vi "CANOpen NMTs.vi"(8 "error in (no error)":errorcluster, 11 "Node Ptr":T3 format="%.0x") -> (0 "error out":errorcluster)   [LabVIEW 2021, in "CANOpen Addon System Explorer.lvlib"]
uses:
  CANOpen Addon System Explorer.lvlib
  <vilib>/NI VeriStand/Custom Device API/Custom Device Item Ref.ctl
  Driver/Async VIs/CANOpen_Main/SubVIs/CanOpen_NMT_Config.ctl
  Driver/Async VIs/CANOpen_Main/SubVIs/CanOpen_NMT_Static detect.ctl
  Shared/CANOpen Addon GUID Lookup Global.vi
  <vilib>/NI VeriStand/Custom Device API/Get Item Property (Variant).vi
  <vilib>/NI VeriStand/Custom Device API/Set Item Property (Variant).vi
  <vilib>/NI VeriStand/Custom Device API/Custom Device API.lvlib
  Shared/CANOpen Addon Shared.lvlib
  Driver/CANOpen Addon Engine.lvlib
panel:
  in  "*HB NG":T1={"Mode"=enum."HB", "Update Time"=100, "Static detect in None"=enum."NG"} caption="Hearbeat and Node Guarding settings"
  in  "*Stop and Reset on Shutdown":bool=TRUE caption="Stop and Reset node on Shutdown"
  in  "*Emergency":bool=TRUE caption="Emergency enabled"
  in  "*Delay for opp. state (ms)":dbl=100.0 caption="Delay (ms) before going to run mode"
  in  "*Node init static SDO state":u16(ring)=128 caption="Inital mode before configuration" items=["start remote node"=1, "enter pre-operational"=128]
  in  "*Node run state":u16(ring)=1 caption="Mode in run state" items=["start remote node"=1, "stop remote node"=2, "enter pre-operational"=128, "reset node"=129, "reset communication"=130]
  in  "SHDocVw.IWebBrowser2":refnum<k7>(container)
  in  "Header":cluster{"Section Name":string}={"Section Name"="NMT"}
  in  "Description":string
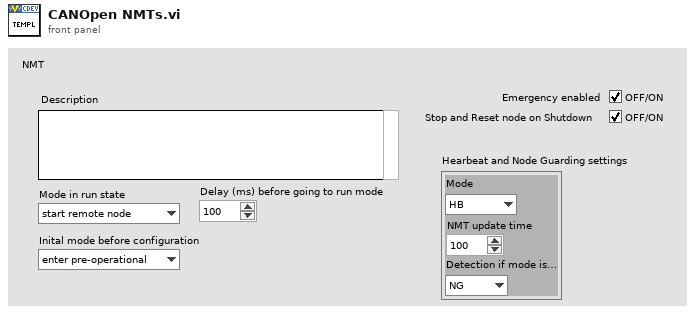
[diagram p1: front panel]
types:
  T1 = typedef "CANOpen Addon Engine.lvlib/CanOpen_NMT_Config.ctl" = cluster{"Mode":T2, "Update Time":u16, "Static detect in None":T2}
  T2 = typedef "CANOpen Addon Engine.lvlib/CanOpen_NMT_Static detect.ctl" = enum16{"None", "HB", "NG"}
  T3 = typedef "Custom Device API.lvlib/Custom Device Item Ref.ctl" = u64
  T4 = typedef "Custom Device API.lvlib/Custom Device Commands.ctl" = enum16{"Default", "Item renamed", "Shutdown", "Dynamic button pressed"}
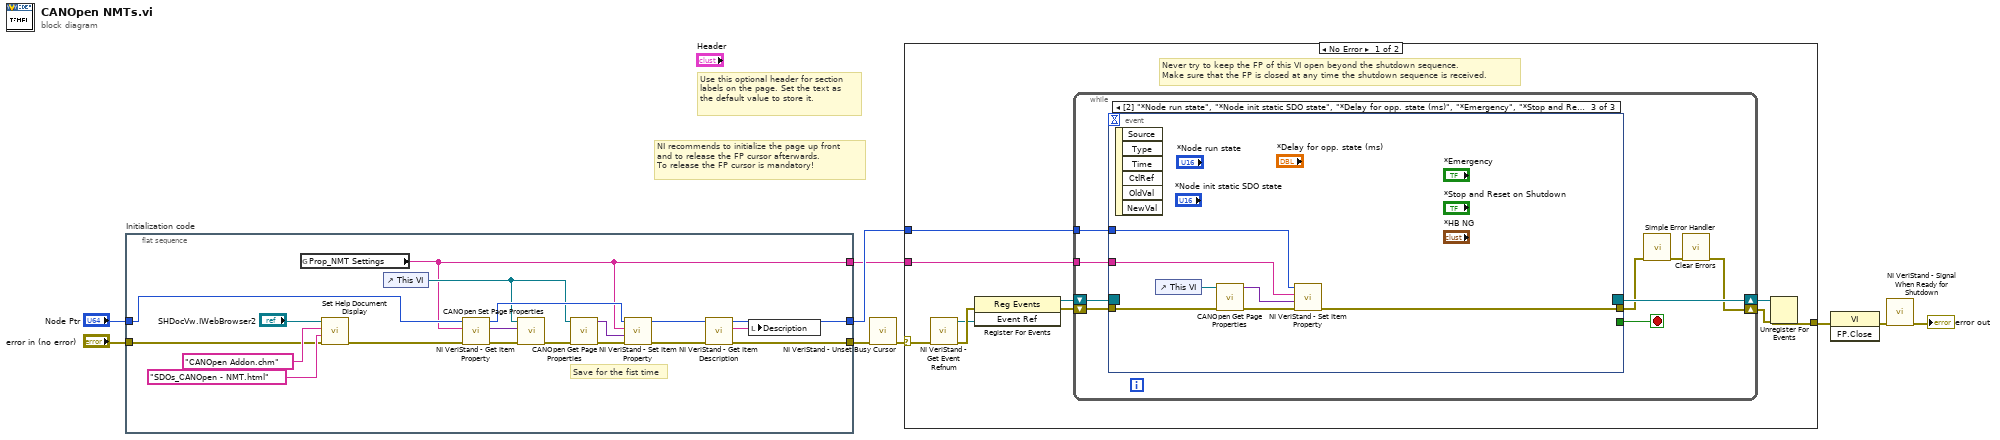
[diagram p0: block diagram]
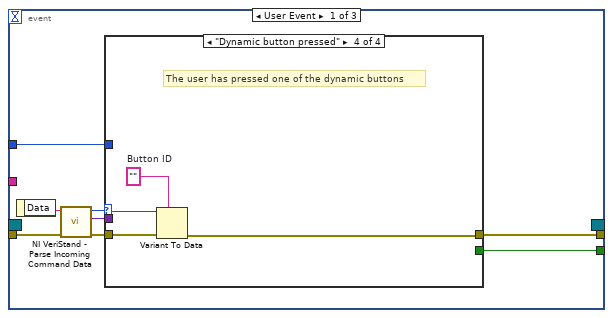
[diagram p2: hidden frame]
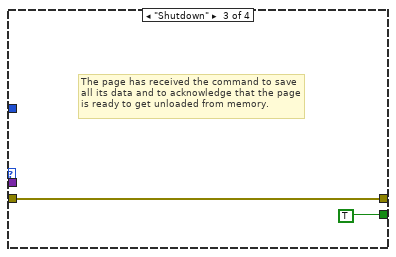
[diagram p5: hidden frame]
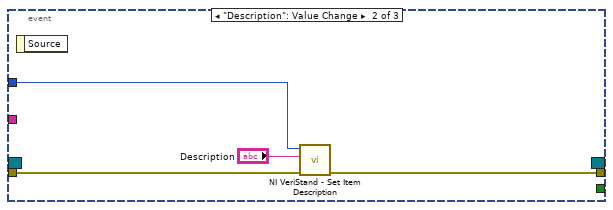
[diagram p6: hidden frame]
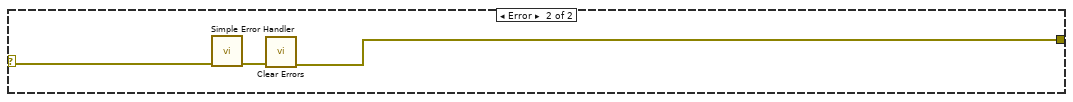
[diagram p7: hidden frame]
diagram:
  # "Use this optional header for section labels on the page. Set the text as the default value to store it."
  # "NI recommends to initialize the page up front\nand to release the FP cursor afterwards.\nTo release the FP cursor is mandatory!"
  n1 = flat-sequence "Initialization code" {
    tunnel: "error in (no error)" -> [w24]
    tunnel: "Node Ptr" -> [w14]
    tunnel: [w23] -> w5
    tunnel: [w22] -> w2
    tunnel: [w10] -> w1
    frame #0 {
      # "Save for the fist time"
      n2 = global read "CANOpen Addon GUID Lookup Global.vi" "Prop_NMT Settings"() -> (w10:string)
      n3 = call "Set Help Document Display.vi"("error in (no error)"=w24, "HTML File"="SDOs_CANOpen - NMT.html", "Main CHM File"="CANOpen Addon.chm", "SHDocVw.IWebBrowser2"="SHDocVw.IWebBrowser2") -> ("error out"=w11:errorcluster)  [unwired: 7 in]
      n4 = control-ref of="This VI"() -> (w20:refnum<vi>)
      n5 = call-poly <vilib>:"NI VeriStand - Get Item Property.vi"("error in (no error)"=w11, "Property Name"=w10, "Item Ref in"=w14) -> ("error out"=w15:errorcluster, "Value"=w16:variant, "Item Ref out"=w21:T3)  [unwired: 5 in, 1 out]
      n6 = call "CANOpen Set Page Properties.vi"("error in"=w15, "variant"=w16, "This VI"=w20) -> ("error out"=w19:errorcluster)  [unwired: 8 in]
      n7 = call "CANOpen Get Page Properties.vi"("error in (no error)"=w19, "This VI"=w20) -> ("error out"=w17:errorcluster, "Settings"=w18:variant)  [unwired: 8 in]
      n8 = call-poly <vilib>:"NI VeriStand - Set Item Property.vi"("error in (no error)"=w17, "Value"=w18, "Property Name"=w10, "Item Ref in"=w21) -> ("error out"=w12:errorcluster, "Item Ref out"=w13:T3)  [unwired: 5 in, 1 out]
      n9 = call <vilib>:"NI VeriStand - Get Item Description.vi"("error in (no error)"=w12, "Item Ref in"=w13) -> ("error out"=w23:errorcluster, "Description"=w28:string, "Item Ref out"=w22:T3)  [unwired: 7 out]
      n10 = local write "Description"(w28) -> ()
    }
  }
  n11 = call <vilib>:"NI VeriStand - Unset Busy Cursor.vi"("error in (no error)"=w5) -> ("error out"=w4:errorcluster)  [unwired: 10 out]
  n12 = case shown="No Error" w4 {
    selector: w4 -> [w30 w77]
    tunnel: [w35 w75] -> w9
    tunnel: w2 -> [w31 _]
    tunnel: w1 -> [w29 _]
    frame No Error {
      # "Never try to keep the FP of this VI open beyond the shutdown sequence.\nMake sure that the FP is closed at any time the shutdown sequence is received."
      n13 = call <vilib>:"NI VeriStand - Get Event Refnum.vi"("error in (no error)"=w30) -> ("error out"=w38:errorcluster, "Event Ref"=w34:refnum<user-event>)  [unwired: 9 out]
      n14 = register-events(error in=w38, w34) -> (reference out=w32:refnum<event-registration>, error out=w33:errorcluster)  [unwired: 1 in]
      n15 = while {
        tunnel: w31 -> [w43]
        shift-right: [w40] -> w36
        shift-left: w33 -> [w46]
        shift-right: [w47] -> w37
        shift-left: w32 -> [w45]
        tunnel: w29 -> [w39]
        stop <- w44 stop-if-true
        n16 = event shown="[2] \"*Node run state\", \"*Node init static SDO state\", \"*Delay for opp. state (ms)\", \"*Emergency\", \"*Stop and Reset on Shutdown\", \"*HB NG\": Value Change" {
          selector: w45 -> [_ _ _]
          dyn-events: [_ _ _] -> w47
          timeout: _ -> [_ _ _]
          tunnel: w46 -> [w55 w66 w72]
          tunnel: [w51 _ _] -> w44
          tunnel: [w50 w65 w69] -> w42
          tunnel: w43 -> [w49 w67 w71]
          tunnel: w39 -> [_ _ w70]
          event User Event {
            n17 = event-data() -> ("Data"=w54:string)  [unwired: 1 out]
            n18 = call <vilib>:"NI VeriStand - Parse Incoming Command Data.vi"("error in (no error)"=w55, "Incoming data"=w54) -> ("error out"=w53:errorcluster, "Outgoing data"=w48:variant, "Action"=w52:T4)  [unwired: 7 out]
            n19 = case shown="\"Dynamic button pressed\"" w52 {
              tunnel: w53 -> [w56 w57 w58 w63]
              tunnel: [_ _ TRUE _] -> w51
              tunnel: [w56 w57 w58 w60] -> w50
              tunnel: w49 -> [_ _ _ _]
              tunnel: w48 -> [_ _ _ w62]
              frame "Default", Default {
              }
              frame "Item renamed" {
              }
              frame "Shutdown" {
                # "The page has received the command to save all its data and to acknowledge that the page is ready to get unloaded from memory."
              }
              frame "Dynamic button pressed" {
                w61 = ""  # Button ID
                # "The user has pressed one of the dynamic buttons"
                n20 = Variant To Data(error in=w63, type=w61, Variant=w62) -> (error out=w60:errorcluster)  [unwired: 1 out]
              }
            }
          }
          event "Description": Value Change {
            n21 = event-data() -> ()  [unwired: 2 out]
            n22 = call <vilib>:"NI VeriStand - Set Item Description.vi"("error in (no error)"=w66, "Description"="Description", "Item Ref in"=w67) -> ("error out"=w65:errorcluster)  [unwired: 8 out]
          }
          event "*Node run state", "*Node init static SDO state", "*Delay for opp. state (ms)", "*Emergency", "*Stop and Reset on Shutdown": Value Change {
            n23 = event-data() -> ()  [unwired: 7 out]
            n24 = control-ref of="This VI"() -> (w68:refnum<vi>)
            n25 = call "CANOpen Get Page Properties.vi"("error in (no error)"=w72, "This VI"=w68) -> ("error out"=w74:errorcluster, "Settings"=w73:variant)  [unwired: 8 in]
            n26 = call-poly <vilib>:"NI VeriStand - Set Item Property.vi"("error in (no error)"=w74, "Value"=w73, "Property Name"=w70, "Item Ref in"=w71) -> ("error out"=w69:errorcluster)  [unwired: 5 in, 2 out]
          }
        }
        n27 = call <vilib>:"Simple Error Handler.vi"("error in (no error)"=w42) -> ("error out"=w41:errorcluster)  [unwired: 1 in, 7 out]
        n28 = call <vilib>:"Clear Errors.vi"("error in (no error)"=w41) -> ("error out"=w40:errorcluster)  [unwired: 1 in, 5 out]
      }
      n29 = Unregister For Events(event registration refnum=w37, error in=w36) -> (error out=w35:errorcluster)
    }
    frame Error {
      n30 = call <vilib>:"Simple Error Handler.vi"("error in (no error)"=w77) -> ("error out"=w76:errorcluster)  [unwired: 1 in, 7 out]
      n31 = call <vilib>:"Clear Errors.vi"("error in (no error)"=w76) -> ("error out"=w75:errorcluster)  [unwired: 1 in, 5 out]
    }
  }
  n32 = invoke class="VI" method="FP.Close"(error in=w9) -> (error out=w8:errorcluster)  [unwired: 2 in, 2 out]
  n33 = call <vilib>:"NI VeriStand - Signal When Ready for Shutdown.vi"("error in (no error)"=w8) -> ("error out"=→"error out":errorcluster)  [unwired: 10 out]
